vi "Read One Config Key.vi"(8 "error in (no error)":errorcluster, 9 "key":string, 10 "default value":string, 11 "Refnum in":T1) -> (0 "error out":errorcluster, 2 "value":string, 3 "Refnum out":T1)   [LabVIEW 2018, in "Air Cooler Application.lvlib" / "Air Cooler Application.lvclass"]
doc: "Read one key from the config file."
uses:
  Air Cooler Application.lvclass
  <vilib>/Utility/config.llb/Config Data RefNum.ctl
  <vilib>/Utility/config.llb/Read Key (String).vi
  <vilib>/Utility/config.llb/NI_LVConfig.lvlib
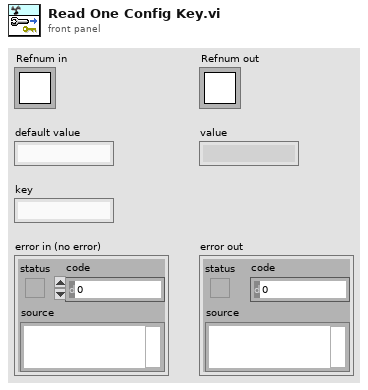
[diagram p1: front panel]
types:
  T1 = typedef "NI_LVConfig.lvlib/Config Data RefNum.ctl" = refnum<k1>
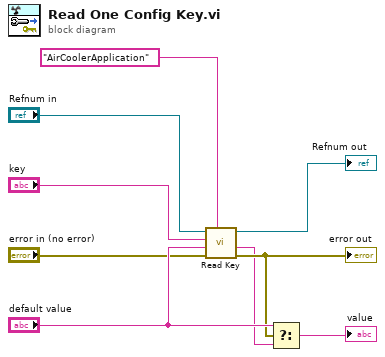
[diagram p0: block diagram]
diagram:
  n1 = call-poly <vilib>:"Read Key.vi"("section"="AirCoolerApplication", "error in (no error)"="error in (no error)", "default value"="default value", "key"="key", "refnum"="Refnum in") -> ("error out"=w6:errorcluster, "value"=w4:string, "refnum out"=→"Refnum out":T1)  [unwired: 3 in, 1 out]
  "error out" <- w6
  n2 = Select(t="default value", s=w6, f=w4) -> (s? t:f=→"value":string)
